vi "Detect QR Codes.vi"   [LabVIEW 2020, in "feature_detection.lvlib" / "QR Code Detector.lvclass"]
uses:
  QR Code Detector.lvclass
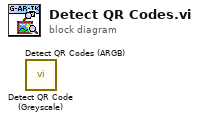
[diagram p0: block diagram]
diagram:
  n1 = call "Detect QR Code (Greyscale).vi"() -> ()  [unwired: 9 in, 3 out]
  n2 = call "Detect QR Codes (ARGB).vi"() -> ()  [unwired: 9 in, 3 out]
